vi "Usermgt.vi"(8 "error In":errorcluster) -> (0 "error out":errorcluster)   [LabVIEW 2015]
uses:
  Um- Save.ctl
  Um-Delete.ctl
  Um-Exit.ctl
  <vilib>/addons/database/Connection.llb/DB Tools Open Connec (String).vi
  <vilib>/addons/database/_DB Variant To Data/Database Variant To Data.xnode
  <vilib>/addons/database/NI_Database_API.lvlib
panel:
  out "User Name 2":string
  out "error out 2":errorcluster
  in  "Exit":T1
  in  "Deleat":T2
  in  "Save":T3
  in  "User Type":string
  in  "User Type":u16(ring) items=["Operator", "Supervisor", "admin"]
  in  "Re-Password":string
  in  "Password":string
  in  "User Name":string
  in  "User Table":i32(listbox)
  # "User Create"
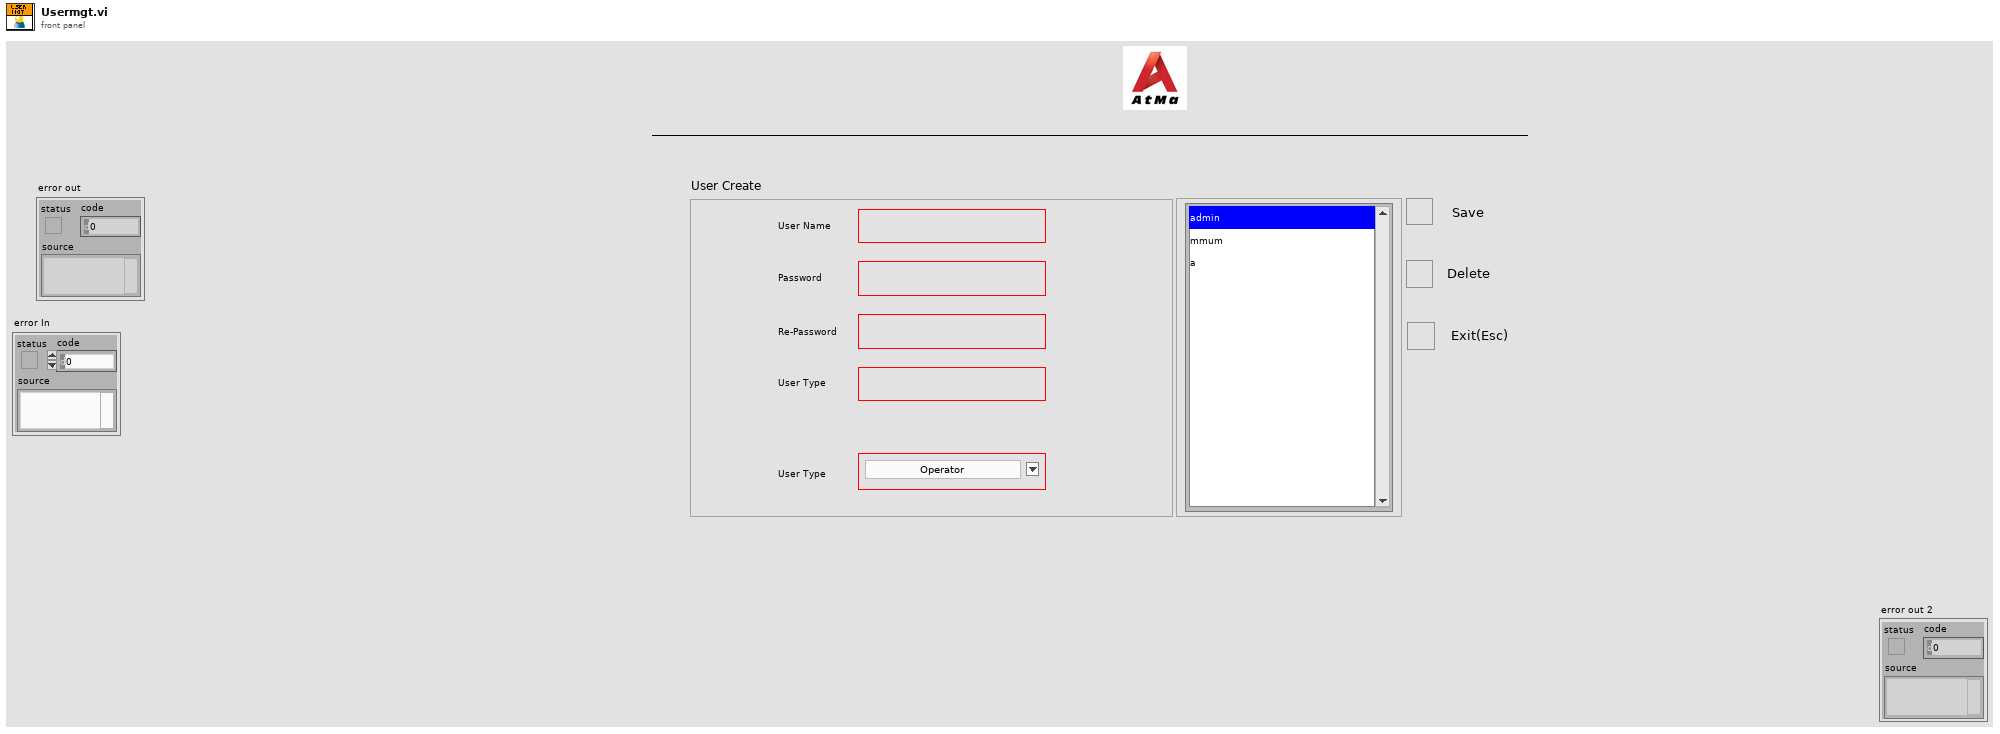
[diagram p1: front panel]
types:
  T1 = typedef "Um-Exit.ctl" = bool
  T2 = typedef "Um-Delete.ctl" = bool
  T3 = typedef "Um- Save.ctl" = bool
  T4 = cluster{"User Name":string, "Password":string, "User Type":string}
  T5 = typedef "NI_Database_API.lvlib/Conn ObjectReference.ctl" = refnum<k1>
  T6 = cluster{"User Name":string, "Password":string, "User Type":string, "Access right":string}
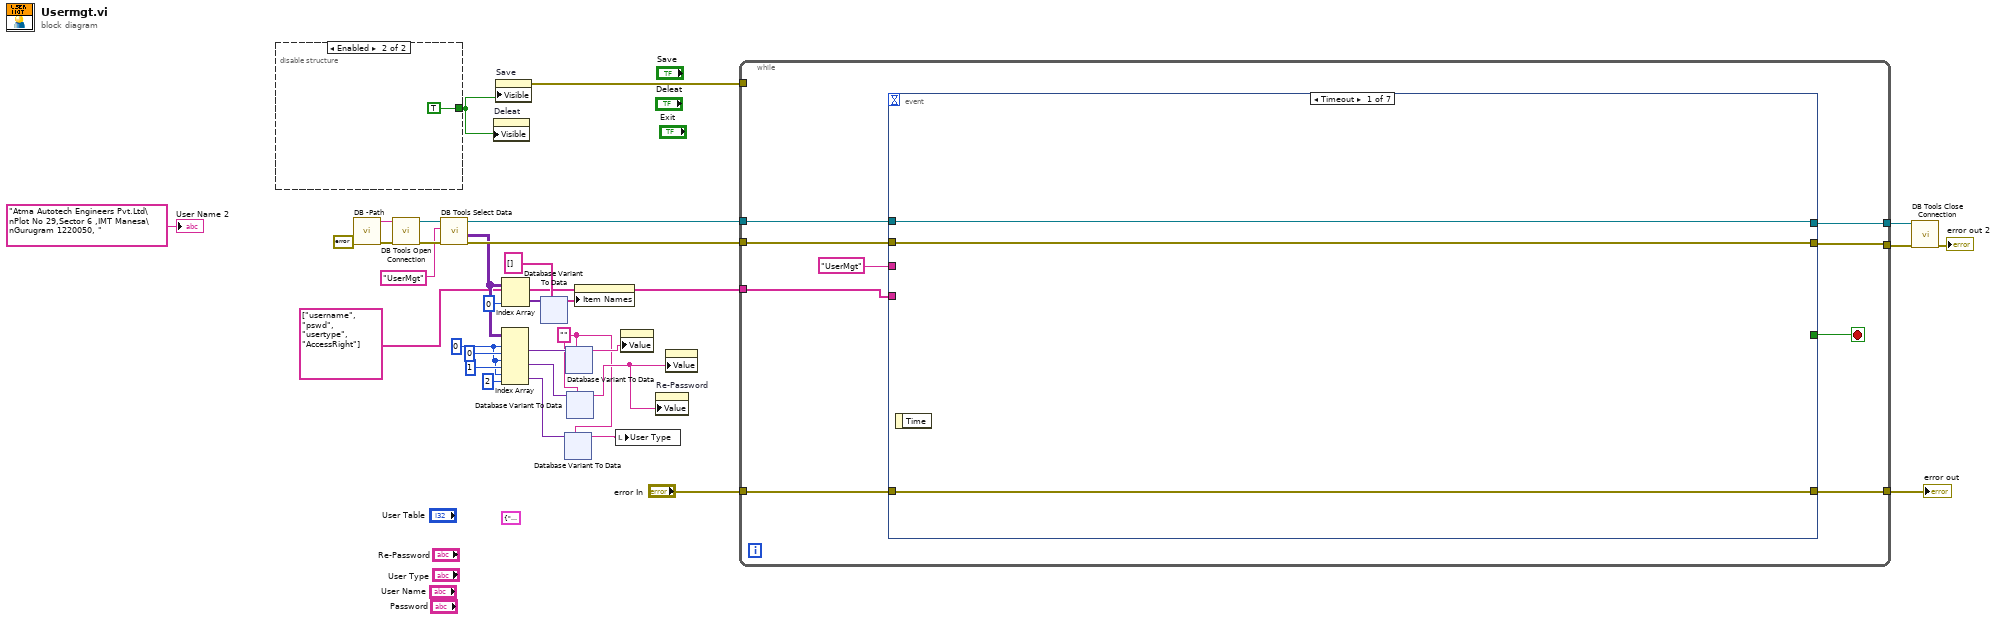
[diagram p0: block diagram]
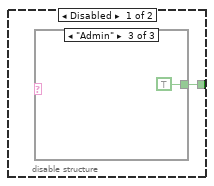
[diagram p2: hidden frame]
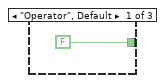
[diagram p3: hidden frame]
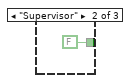
[diagram p4: hidden frame]
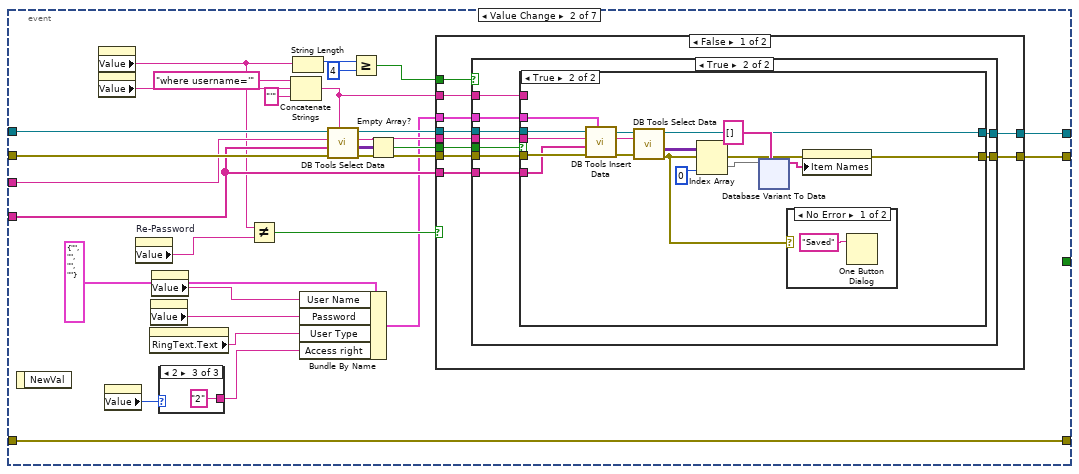
[diagram p5: hidden frame]
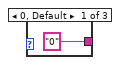
[diagram p6: hidden frame]
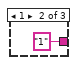
[diagram p7: hidden frame]
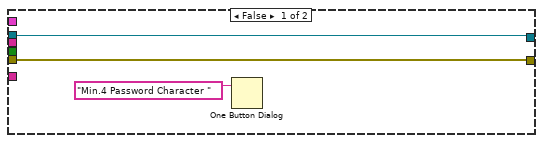
[diagram p8: hidden frame]
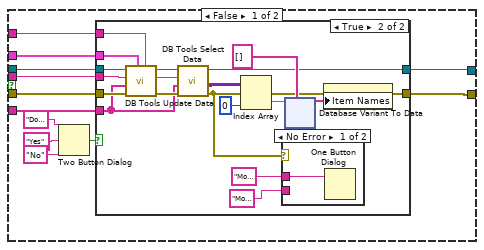
[diagram p9: hidden frame]
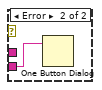
[diagram p11: hidden frame]
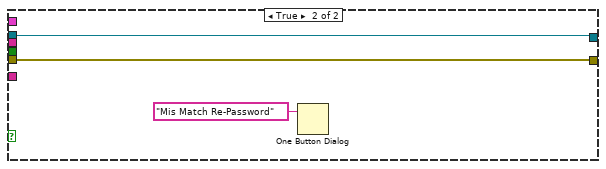
[diagram p13: hidden frame]
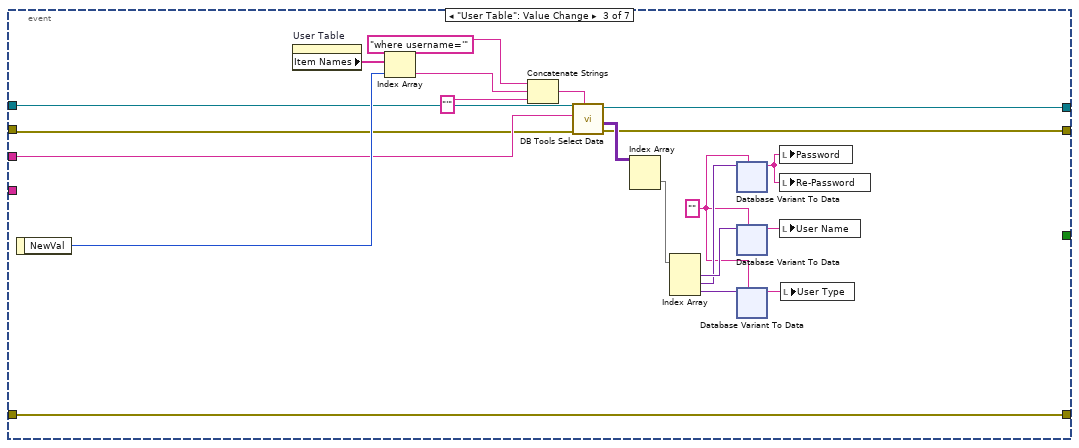
[diagram p14: hidden frame]
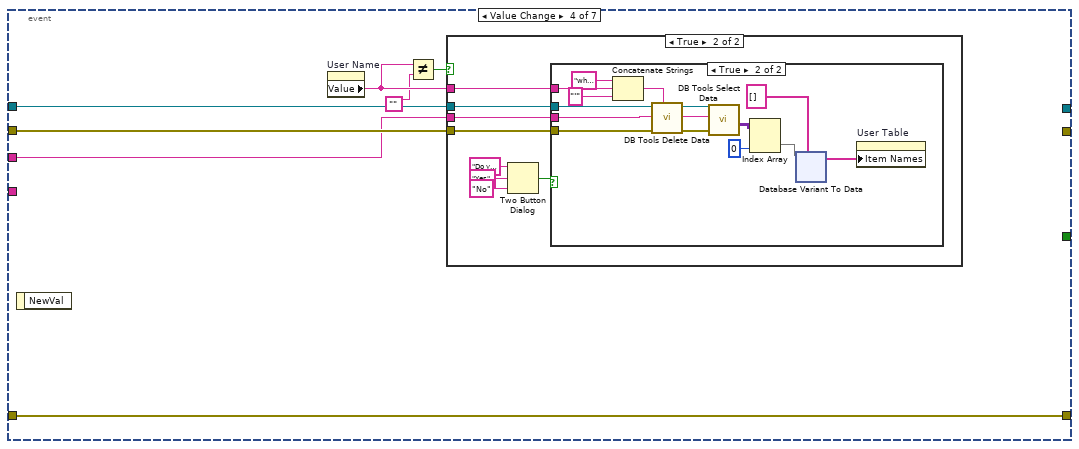
[diagram p15: hidden frame]
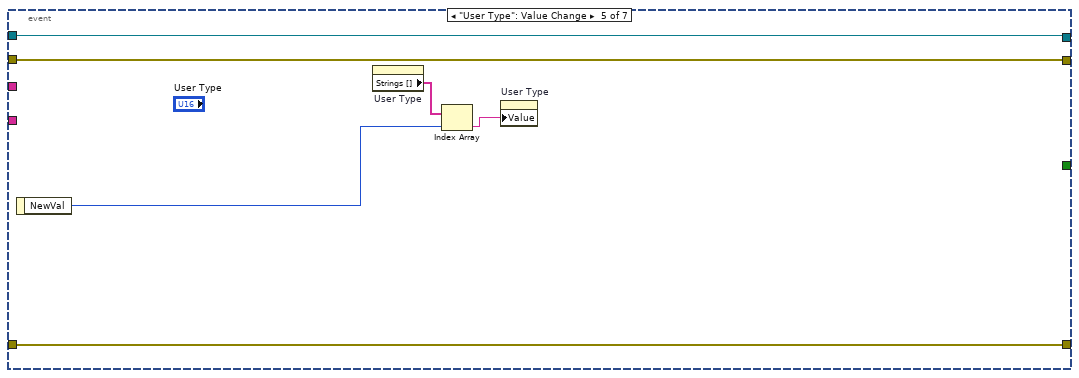
[diagram p18: hidden frame]
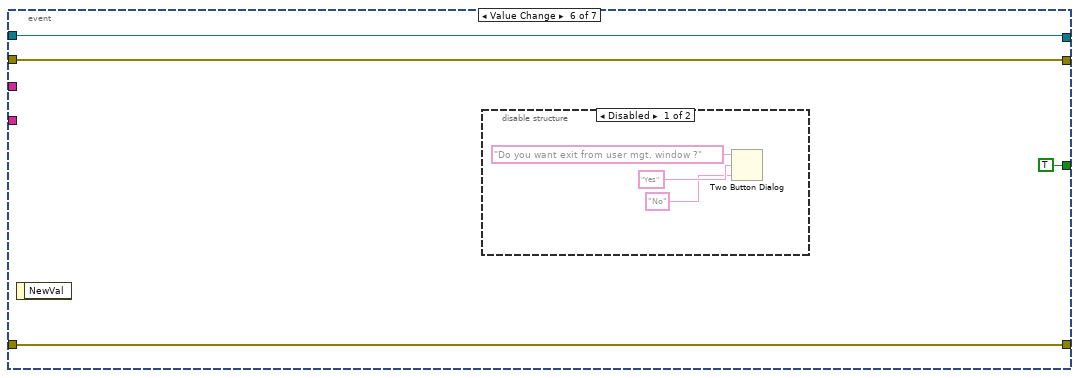
[diagram p19: hidden frame]
diagram:
  w13 = ""
  w12 = 0 ("index (row)")
  (unwired) T4 {"User Name"="", "Password"="", "User Type"=""} ("Input data")
  n1 = disable-structure shown="Enabled" {
    disable-tunnel: [w33 TRUE] -> w8
    frame Disabled {
      n2 = case shown="\"Admin\"" {
        selector: _ -> [_ _ _]
        tunnel: [FALSE FALSE TRUE] -> w33
        frame "Operator", Default {
        }
        frame "Supervisor" {
        }
        frame "Admin" {
        }
      }
    }
    frame Enabled {
    }
  }
  n3 = call "DB -Path.vi"() -> ("String"=w32:string)  [unwired: 11 in]
  n4 = call-poly <vilib>:"DB Tools Open Connection.vi"("error in (no error)"=errorcluster {"status"=FALSE, "code"=0, "source"=""}, "connection information"=w32) -> ("error out"=w29:errorcluster, "connection reference"=w28:T5)  [unwired: 6 in]
  n5 = call <vilib>:"DB Tools Select Data.vi"("error in (no error)"=w29, "table"="UserMgt", "connection reference"=w28) -> ("error out"=w26:errorcluster, "data"=w19:variant[][], "connection reference out"=w27:T5)  [unwired: 3 in]
  n6 = property on="Deleat" class="Bool (strict)"("Visible"=w8) -> ()  [unwired: 2 in, 2 out]
  n7 = property on="Save" class="Bool (strict)"("Visible"=w8) -> (error out=w7:errorcluster)  [unwired: 2 in, 1 out]
  n8 = Index Array(array=w19, index (row) #1=w12, index (col) #1=0 ("disabled index (col)"), index (row) #2=w12, index (col) #2=1 ("disabled index (col)"), index (row) #3=w12, index (col) #3=2 ("disabled index (col)")) -> (element #1=w20:variant, element #2=w16:variant, element #3=w10:variant)
  n9 = Index Array(array=w19, index (col)=0 ("disabled index (col)")) -> (element=w24:variant[])  [unwired: 1 in]
  n10 = xnode "Database Variant To Data"("database variant"=w24, "type"=string[] []) -> ("data"=w21:string[])  [unwired: 1 in, 1 out]
  n11 = xnode "Database Variant To Data"("database variant"=w10, "type"=w13) -> ("data"=w9:string)  [unwired: 1 in, 1 out]
  n12 = xnode "Database Variant To Data"("database variant"=w20, "type"=w13) -> ("data"=w15:string)  [unwired: 1 in, 1 out]
  n13 = xnode "Database Variant To Data"("database variant"=w16, "type"=w13) -> ("data"=w14:string)  [unwired: 1 in, 1 out]
  n14 = property on="User Table" class="LstBox (strict)"("Item Names"=w21) -> ()  [unwired: 2 in, 2 out]
  n15 = local write "User Type"(w9) -> ()
  n16 = property on="User Name" class="Str"("Value"=w15) -> ()  [unwired: 2 in, 2 out]
  n17 = property on="Re-Password" class="Str"("Value"=w14) -> ()  [unwired: 2 in, 2 out]
  n18 = property on="Password" class="Str"("Value"=w14) -> ()  [unwired: 2 in, 2 out]
  n19 = while {
    tunnel: w27 -> [w45]
    tunnel: w26 -> [w44]
    tunnel: [w42] -> w31
    tunnel: [w41] -> w30
    tunnel: w7 -> [_]
    tunnel: string[] ["username", "pswd", "usertype", "AccessRight"] ("columns") -> [w40]
    tunnel: "error In" -> [w39]
    tunnel: [w38] -> w3
    stop <- w46 stop-if-true
    n20 = event shown="[0] Timeout" {
      selector: _ -> [_ _ _ _ _ _ _]
      dyn-events: _ -> [_ _ _ _ _ _ _]
      timeout: _ -> [_ _ _ _ _ _ _]
      tunnel: [_ _ _ _ _ TRUE ("T button?") _] -> w46
      tunnel: w45 -> [w49 w77 w236 w353 w416 w423 _]
      tunnel: w44 -> [w48 w76 w235 w352 w415 w422 _]
      tunnel: "UserMgt" ("table") -> [_ w69 w244 w348 _ _ _]
      tunnel: w40 -> [_ w68 _ _ _ _ _]
      tunnel: [w49 w67 w234 _ w416 w423 _] -> w42
      tunnel: [w48 w66 w233 _ w415 w422 _] -> w41
      tunnel: w39 -> [w47 w50 w230 w347 w414 w420 w427]
      tunnel: [w47 w50 w230 w347 w414 w420 w427] -> w38
      event Timeout {
        n21 = event-data() -> ()  [unwired: 1 in, 1 out]
      }
      event Value Change {
        n22 = event-data() -> ()  [unwired: 1 in, 1 out]
        n23 = property on="Password" class="Str"() -> ("Value"=w52:string)  [unwired: 2 in, 2 out]
        n24 = property on="User Name" class="Str"() -> ("Value"=w51:string)  [unwired: 2 in, 2 out]
        n25 = property on="User Table" class="LstBox (strict)"() -> ("Value"=w55:i32)  [unwired: 2 in, 2 out]
        n26 = property on="Re-Password" class="Str"() -> ("Value"=w60:string)  [unwired: 2 in, 2 out]
        n27 = property on="User Type" class="Ring (strict)"() -> ("RingText.Text"=w57:string)  [unwired: 2 in, 2 out]
        n28 = property on="Password" class="Str"() -> ("Value"=w59:string)  [unwired: 2 in, 2 out]
        n29 = property on="User Name" class="Str"() -> ("Value"=w58:string)  [unwired: 2 in, 2 out]
        n30 = case shown="2" w55 {
          tunnel: ["0" "1" "2"] -> w54
          frame 0, Default {
          }
          frame 1 {
          }
          frame 2 {
          }
        }
        n31 = Not Equal?(x=w52, y=w60) -> (x != y?=w61:bool)
        n32 = Concatenate Strings("where username='" ("condition"), w51, "'" ("User Name")) -> (w65:string)
        n33 = String Length(string=w52) -> (length=w64:i32)
        n34 = Bundle By Name(cluster=T6 {"User Name"="", "Password"="", "User Type"="", "Access right"=""} ("input cluster"), "User Name"=w58, "Password"=w59, "User Type"=w57, "Access right"=w54) -> (w53:T6)
        n35 = call <vilib>:"DB Tools Select Data.vi"("condition"=w65, "error in (no error)"=w76, "columns"=w68, "table"=w69, "connection reference"=w77) -> ("error out"=w70:errorcluster, "data"=w75:variant[][], "connection reference out"=w71:T5)  [unwired: 1 in]
        n36 = Greater Or Equal?(x=w64, y=4) -> (x >= y?=w62:bool)
        n37 = Empty Array?(array=w75) -> (empty?=w74:bool)
        n38 = case shown="False" w61 {
          tunnel: w74 -> [w90 _]
          tunnel: w71 -> [w89 w229]
          tunnel: w70 -> [w88 w228]
          tunnel: w69 -> [w87 _]
          tunnel: w68 -> [w86 _]
          tunnel: w53 -> [w85 _]
          tunnel: [w84 w229] -> w67
          tunnel: [w83 w228] -> w66
          tunnel: w65 -> [w82 _]
          tunnel: w62 -> [w81 _]
          frame False {
            n39 = case shown="True" w81 {
              tunnel: w90 -> [_ w102]
              tunnel: w89 -> [w93 w101]
              tunnel: w88 -> [w92 w100]
              tunnel: w87 -> [_ w99]
              tunnel: w86 -> [_ w98]
              tunnel: w85 -> [_ w97]
              tunnel: [w93 w96] -> w84
              tunnel: [w92 w95] -> w83
              tunnel: w82 -> [_ w94]
              frame False {
                n40 = One Button Dialog(message="Min.4 Password Character ") -> ()  [unwired: 1 in, 1 out]
              }
              frame True {
                n41 = case shown="True" w102 {
                  tunnel: w101 -> [w114 w187]
                  tunnel: w100 -> [w113 w186]
                  tunnel: w99 -> [w108 w181]
                  tunnel: w98 -> [w105 w185]
                  tunnel: w97 -> [w106 w184]
                  tunnel: [w104 w175] -> w96
                  tunnel: [w103 w174] -> w95
                  tunnel: w94 -> [w107 _]
                  frame False {
                    n42 = Two Button Dialog(message="Do you want  modification" ("T button name (\"OK\")"), 1:"No" ("F button name (\"Cancel\")"), 2:"Yes" ("T button name (\"OK\")")) -> (T button?=w112:bool)
                    n43 = case shown="True" w112 {
                      tunnel: w114 -> [w116 w133]
                      tunnel: w113 -> [w115 w132]
                      tunnel: w108 -> [_ w127]
                      tunnel: w107 -> [_ w131]
                      tunnel: w106 -> [_ w130]
                      tunnel: w105 -> [_ w121]
                      tunnel: [w116 w120] -> w104
                      tunnel: [w115 w119] -> w103
                      frame False {
                      }
                      frame True {
                        n44 = call <vilib>:"DB Tools Update Data.vi"("condition"=w131, "data"=w130, "error in (no error)"=w132, "columns"=w121, "table"=w127, "connection reference"=w133) -> ("error out"=w128:errorcluster, "connection reference out"=w129:T5)  [unwired: 4 in]
                        n45 = call <vilib>:"DB Tools Select Data.vi"("error in (no error)"=w128, "columns"=w121, "table"=w127, "connection reference"=w129) -> ("error out"=w119:errorcluster, "data"=w126:variant[][], "connection reference out"=w120:T5)  [unwired: 2 in]
                        n46 = Index Array(array=w126, index (col)=0 ("disabled index (col)")) -> (element=w124:variant[])  [unwired: 1 in]
                        n47 = case shown="No Error" w119 {
                          tunnel: "Modification is Successfully" ("T button name (\"OK\")") -> [w134 _]
                          tunnel: "Modification is Unsuccessfully" ("T button name (\"OK\")") -> [_ w135]
                          frame No Error {
                            n48 = One Button Dialog(message=w134) -> ()  [unwired: 1 in, 1 out]
                          }
                          frame Error {
                            n49 = One Button Dialog(message=w135) -> ()  [unwired: 1 in, 1 out]
                          }
                        }
                        n50 = xnode "Database Variant To Data"("database variant"=w124, "type"=string[] []) -> ("data"=w122:string[])  [unwired: 1 in, 1 out]
                        n51 = property on="User Table" class="LstBox (strict)"("Item Names"=w122) -> ()  [unwired: 2 in, 2 out]
                      }
                    }
                  }
                  frame True {
                    n52 = call <vilib>:"DB Tools Insert Data.vi"("data"=w184, "error in (no error)"=w186, "columns"=w185, "table"=w181, "connection reference"=w187) -> ("error out"=w182:errorcluster, "connection reference out"=w183:T5)  [unwired: 5 in]
                    n53 = call <vilib>:"DB Tools Select Data.vi"("error in (no error)"=w182, "table"=w181, "connection reference"=w183) -> ("error out"=w174:errorcluster, "data"=w180:variant[][], "connection reference out"=w175:T5)  [unwired: 3 in]
                    n54 = Index Array(array=w180, index (col)=0 ("disabled index (col)")) -> (element=w178:variant[])  [unwired: 1 in]
                    n55 = xnode "Database Variant To Data"("database variant"=w178, "type"=string[] []) -> ("data"=w176:string[])  [unwired: 1 in, 1 out]
                    n56 = case shown="No Error" w174 {
                      frame No Error {
                        n57 = One Button Dialog(message="Saved" ("T button name (\"OK\")")) -> ()  [unwired: 1 in, 1 out]
                      }
                      frame Error {
                      }
                    }
                    n58 = property on="User Table" class="LstBox (strict)"("Item Names"=w176) -> ()  [unwired: 2 in, 2 out]
                  }
                }
              }
            }
          }
          frame True {
            n59 = One Button Dialog(message="Mis Match Re-Password") -> ()  [unwired: 1 in, 1 out]
          }
        }
      }
      event "User Table": Value Change {
        w231 = "" ("table")
        n60 = event-data() -> ("NewVal"=w248:i32)  [unwired: 1 in]
        n61 = property on="User Table" class="LstBox (strict)"() -> ("Item Names"=w249:string[])  [unwired: 2 in, 2 out]
        n62 = Index Array(array=w249, index=w248) -> (element=w246:string)
        n63 = Concatenate Strings("where username='" ("condition"), w246, "'" ("User Name")) -> (w245:string)
        n64 = call <vilib>:"DB Tools Select Data.vi"("condition"=w245, "error in (no error)"=w235, "table"=w244, "connection reference"=w236) -> ("error out"=w233:errorcluster, "data"=w243:variant[][], "connection reference out"=w234:T5)  [unwired: 2 in]
        n65 = Index Array(array=w243) -> (element=w242:variant[])  [unwired: 2 in]
        n66 = Index Array(array=w242) -> (element #1=w241:variant, element #2=w240:variant, element #3=w239:variant)  [unwired: 3 in]
        n67 = xnode "Database Variant To Data"("database variant"=w240, "type"=w231) -> ("data"=w237:string)  [unwired: 1 in, 1 out]
        n68 = xnode "Database Variant To Data"("database variant"=w241, "type"=w231) -> ("data"=w238:string)  [unwired: 1 in, 1 out]
        n69 = xnode "Database Variant To Data"("database variant"=w239, "type"=w231) -> ("data"=w232:string)  [unwired: 1 in, 1 out]
        n70 = local write "Password"(w237) -> ()
        n71 = local write "Re-Password"(w237) -> ()
        n72 = local write "User Name"(w238) -> ()
        n73 = local write "User Type"(w232) -> ()
      }
      event Value Change {
        n74 = event-data() -> ()  [unwired: 1 in, 1 out]
        n75 = property on="User Name" class="Str"() -> ("Value"=w351:string)  [unwired: 2 in, 2 out]
        n76 = Not Equal?(x=w351, y="") -> (x != y?=w349:bool)
        n77 = case shown="True" w349 {
          tunnel: w353 -> [_ w357]
          tunnel: w352 -> [_ w356]
          tunnel: w351 -> [_ w355]
          tunnel: w348 -> [_ w354]
          frame False {
          }
          frame True {
            n78 = Two Button Dialog(message="Do you want delete the user id & password", 1:"No" ("F button name (\"Cancel\")"), 2:"Yes" ("T button name (\"OK\")")) -> (T button?=w358:bool)
            n79 = case shown="True" w358 {
              tunnel: w357 -> [_ w375]
              tunnel: w356 -> [_ w374]
              tunnel: w355 -> [_ w370]
              tunnel: w354 -> [_ w367]
              frame False {
              }
              frame True {
                n80 = Concatenate Strings("where username='" ("condition"), w370, "'" ("User Name")) -> (w371:string)
                n81 = call <vilib>:"DB Tools Delete Data.vi"("condition"=w371, "error in (no error)"=w374, "table"=w367, "connection reference"=w375) -> ("error out"=w368:errorcluster, "connection reference out"=w369:T5)  [unwired: 6 in]
                n82 = call <vilib>:"DB Tools Select Data.vi"("error in (no error)"=w368, "table"=w367, "connection reference"=w369) -> ("data"=w365:variant[][])  [unwired: 3 in, 2 out]
                n83 = Index Array(array=w365, index (col)=0 ("disabled index (col)")) -> (element=w364:variant[])  [unwired: 1 in]
                n84 = xnode "Database Variant To Data"("database variant"=w364, "type"=string[] []) -> ("data"=w362:string[])  [unwired: 1 in, 1 out]
                n85 = property on="User Table" class="LstBox (strict)"("Item Names"=w362) -> ()  [unwired: 2 in, 2 out]
              }
            }
          }
        }
      }
      event "User Type": Value Change {
        n86 = event-data() -> ("NewVal"=w419:u16)  [unwired: 1 in]
        n87 = property on="User Type" class="Ring (strict)"() -> ("Strings []"=w418:string[])  [unwired: 2 in, 2 out]
        n88 = Index Array(array=w418, index=w419) -> (element=w417:string)
        n89 = property on="User Type" class="Str"("Value"=w417) -> ()  [unwired: 2 in, 2 out]
      }
      event Value Change {
        n90 = event-data() -> ()  [unwired: 1 in, 1 out]
        n91 = disable-structure shown="Disabled" {
          frame Disabled {
            n92 = Two Button Dialog(message="Do you want exit from user mgt. window ?", 1:"No" ("F button name (\"Cancel\")"), 2:"Yes" ("T button name (\"OK\")")) -> ()  [unwired: 1 out]
          }
          frame Enabled {
          }
        }
      }
      event Panel Close? {
        n93 = event-data() -> ()  [unwired: 1 in, 3 out]
        n94 = event-data("Discard?"=TRUE) -> ()  [unwired: 1 in, 1 out]
      }
    }
  }
  "error out" <- w3
  n95 = call <vilib>:"DB Tools Close Connection.vi"("error in (no error)"=w30, "connection reference"=w31) -> ("error out"=→"error out 2":errorcluster)  [unwired: 5 in]
  "User Name 2" <- "Atma Autotech Engineers Pvt.Ltd\nPlot No 29,Sector 6 ,IMT Manesa\nGurugram 1220050, " ("string")
